vi "Stop Core.vi"(10 "final error code":i32, 11 "Manager in":refnum<class "Manager.lvclass">) -> (3 "Manager out":refnum<class "Manager.lvclass">)   [LabVIEW 2016, in "Manager.lvlib" / "Manager.lvclass"]
doc: "(<B>Filename</B>: Actor Framework.lvlib:Actor.lvclass:Stop Core.vi)\n\nDefines what the actor does before it stops. Use the <B>final error code</B> input to determine whether the actor shut down in response to an error.\n\nBy default, this method does nothing. A descendant class may override it to define behavior, such as shutting down any processes the actor initiated in its override of the Actor Core method."
uses:
  Manager.lvclass
  Manager.lvclass/Manager.ctl
  <vilib>/ActorFramework/Stop Msg/Stop Msg.lvclass/Stop Msg.ctl
  <vilib>/ActorFramework/Message Enqueuer/Message Enqueuer.lvclass/Message Enqueuer.ctl
  <vilib>/ActorFramework/Stop Msg/Send Emergency Stop.vi
  <vilib>/ActorFramework/Stop Msg/Send Normal Stop.vi
  <vilib>/ActorFramework/Message Enqueuer/Enqueue Critical.vi
  <vilib>/ActorFramework/Message Enqueuer/Enqueue.vi
  <vilib>/ActorFramework/Stop Msg/Stop Msg.lvclass
  C:/Program Files (x86)/National Instruments/LabVIEW 2016/vi.lib/ActorFramework/Message/Message.lvclass
  <vilib>/ActorFramework/Message Priority Queue/Priority Enqueue.vi
  <vilib>/ActorFramework/Actor/Actor.lvclass
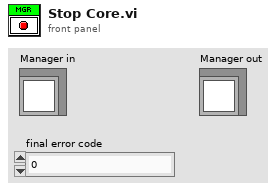
[diagram p1: front panel]
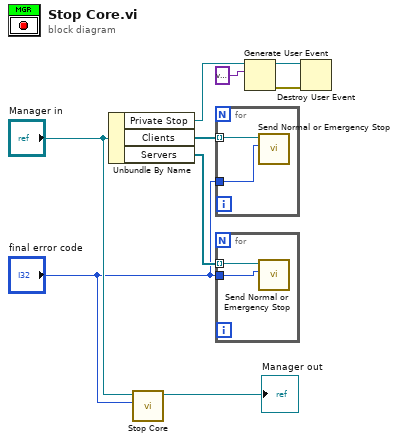
[diagram p0: block diagram]
diagram:
  n1 = Unbundle By Name("Manager in") -> ("Private Stop"=w7:refnum<user-event>, "Clients"=w3:refnum<class "Message Enqueuer.lvclass">[], "Servers"=w2:refnum<class "Message Enqueuer.lvclass">[])
  n2 = call-parent "Stop Core.vi"("final error code"="final error code", "Actor in"="Manager in") -> ("Actor out"=→"Manager out":refnum<class "Manager.lvclass">)  [unwired: 9 in]
  n3 = for {
    tunnel: w3 -> [w11] mode=indexing
    tunnel: "final error code" -> [w10]
    n4 = call <vilib>:"Send Normal or Emergency Stop.vi"("final error code"=w10, "Message Enqueuer"=w11) -> ()  [unwired: 9 in, 1 out]
  }
  n5 = for {
    tunnel: w2 -> [w13] mode=indexing
    tunnel: "final error code" -> [w12]
    n6 = call <vilib>:"Send Normal or Emergency Stop.vi"("final error code"=w12, "Message Enqueuer"=w13) -> ()  [unwired: 9 in, 1 out]
  }
  n7 = Generate User Event(user event=w7, event data cluster=variant ("event data")) -> (user event out=w6:refnum<user-event>, error out=w5:errorcluster)  [unwired: 2 in]
  n8 = Destroy User Event(user event=w6, error in=w5) -> ()  [unwired: 1 out]
